vi "Return Stamp.vi"(8 "error in":errorcluster, 10 "Slot Number":i32, 11 "GrabberTool in":refnum<class "GrabberTool Class.lvclass">) -> (0 "error out":errorcluster, 3 "GrabberTool out":refnum<class "GrabberTool Class.lvclass">)   [LabVIEW 2011, in "GrabberTool Class.lvclass"]
uses:
  GrabberTool Class.lvclass
  Config Manager Class/Type Definitions/Named Position.ctl
  Config Manager Class/Type Definitions/Part Type.ctl
  Config Manager Class/Type Definitions/Offset.ctl
  WorkTable Class/WorkTable Class.lvclass
  Vec3d Class/Vec3d Class.lvclass
  Config Manager Class/Config Manager Class.lvclass
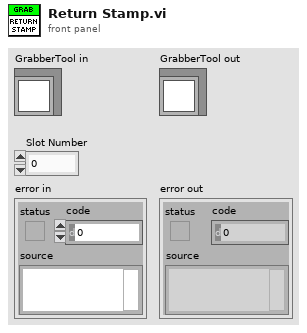
[diagram p1: front panel]
types:
  T1 = typedef "Named Position.ctl" = enum16{"home", "module_chuck_0", "module_chuck_1", "module_chuck_2", "module_chuck_3", "module_chuck_4", "glue_reservoir_chuck", "stamp_tool_chuck", "weight_tool_chuck", "needle_calibration", "tool_rack_pos_0_in", "tool_rack_pos_0_out", "tool_rack_pos_1_in", "tool_rack_pos_1_out", "tool_rack_pos_2_in", "tool_rack_pos_2_out", "front_load_position", "grabber_start_pos", "between_chuck_0_and_1", "between_chuck_2_and_3"}
  T2 = typedef "Part Type.ctl" = enum16{"BBM", "HDI", "BARE HDI", "GLUERESERVOIR", "STAMP_1", "STAMP_2", "STAMP_3", "STAMP_4", "STAMP_5", "WEIGHT_1", "WEIGHT_2", "WEIGHT_3", "WEIGHT_4", "WEIGHT_5", "WEIGHT_6", "WEIGHT_7", "WEIGHT_8", "PICKER_TOOL", "GRABER_TOOL"}
  T3 = typedef "Offset.ctl" = enum16{"needle_offset", "tool_holder_offset"}
  T4 = typedef "Worktable_Stamps.ctl" = cluster{"Stamp Slots":T5[], "Vacuum Channel":i32}
  T5 = typedef "Worktable_Stamp.ctl" = cluster{"Stamp State":enum16{"Empty", "Populated", "Used"}, "Location/Orientation":T6, "Stamp Type":T7}
  T6 = typedef "Position_Orientation.ctl" = cluster{"Center":refnum<class "Vec3d Class.lvclass">, "Orientation":refnum<class "Orient3d Class.lvclass">}
  T7 = typedef "Stamp Type.ctl" = enum16{"Stamp 1", "Stamp 2", "Stamp 3", "Stamp 4", "Stamp 5"}
  T8 = typedef "Gluing Parameters.ctl" = cluster{"Safe Grabber Pickup":dbl, "Safe Grabber Lift":dbl, "Glue Resevoir Wait Time":dbl, "Glue BM Wait Time ":dbl, "Placed Weight X-Move":dbl}
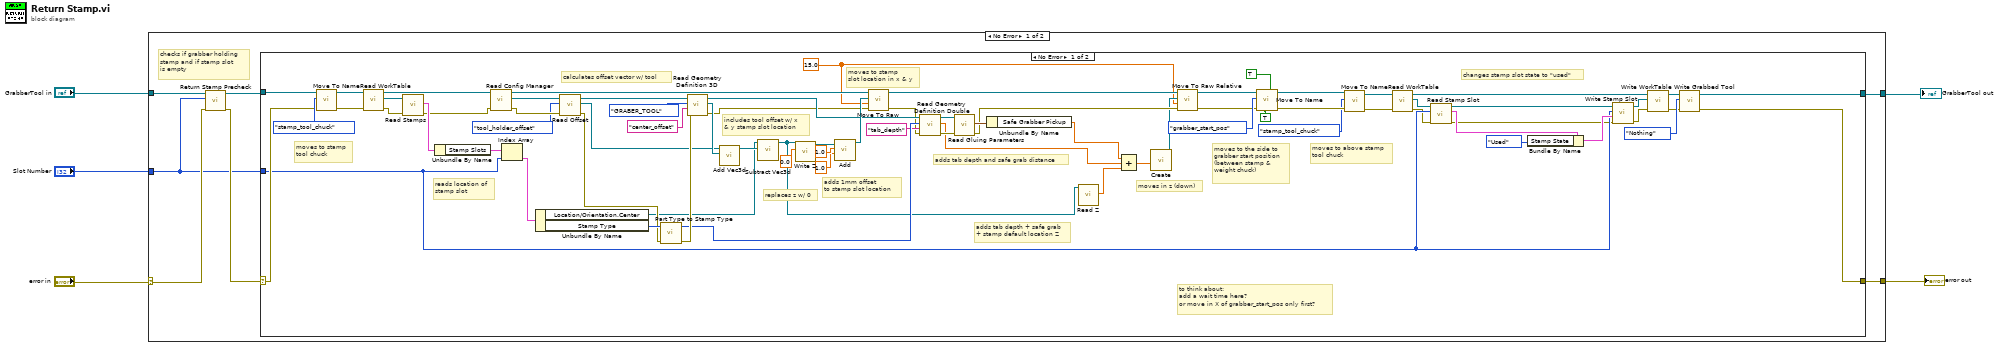
[diagram p0: block diagram]
diagram:
  n1 = case shown="No Error" "error in" {
    selector: "error in" -> [w8 w89]
    tunnel: [w12 w89] -> w5
    tunnel: "GrabberTool in" -> [w10 w90]
    tunnel: "Slot Number" -> [w6 _]
    tunnel: [w11 w90] -> w2
    frame No Error {
      # "checks if grabber holding\nstamp and if stamp slot\nis empty"
      n2 = call "Return Stamp Precheck.vi"("error in (no error)"=w8, "Slot Number"=w6, "GrabberTool Class in"=w10) -> ("error out"=w7:errorcluster, "GrabberTool Class out"=w9:refnum<class "GrabberTool Class.lvclass">)  [unwired: 7 in]
      n3 = case shown="No Error" w7 {
        selector: w7 -> [w83 w88]
        tunnel: [w20 w88] -> w12
        tunnel: w9 -> [w86 w87]
        tunnel: w6 -> [w27 _]
        tunnel: [w21 w87] -> w11
        frame No Error {
          w13 = 15.0 ("Speed")
          # "changes stamp slot state to \"used\""
          # "to think about:\nadd a wait time here?\nor move in X of grabber_start_pos only first?"
          # "moves to above stamp\ntool chuck"
          # "moves to the side to\ngrabber start position\n(between stamp & \nweight chuck)"
          # "moves in z (down)"
          # "adds tab depth + safe grab\n+ stamp default location Z"
          # "adds tab depth and safe grab distance"
          # "moves to stamp\nslot location in x & y"
          # "adds 1mm offset\nto stamp slot location"
          # "includes tool offset w/ x \n& y stamp slot location"
          # "replaces z w/ 0"
          # "calculates offset vector w/ tool"
          # "reads location of\nstamp slot"
          # "moves to stamp\ntool chuck"
          n4 = call-dynamic "Move To Name.vi"("error in"=w83, "Destination"=Named_Position."stamp_tool_chuck", "Gantry in"=w86) -> ("error out"=w82:errorcluster, "Gantry out"=w84:refnum<class "GrabberTool Class.lvclass">)  [unwired: 7 in]
          n5 = call-dynamic "Read WorkTable.vi"("error in"=w82, "Gantry Class in"=w84) -> ("error out"=w80:errorcluster, "WorkTable Class.lvclass"=w81:refnum<class "WorkTable Class.lvclass">, "Gantry Class out"=w76:refnum<class "GrabberTool Class.lvclass">)  [unwired: 7 in]
          n6 = call-dynamic "Read Stamps.vi"("error in (no error)"=w80, "WorkTable Class in"=w81) -> ("error out"=w75:errorcluster, "Stamps"=w79:T4)  [unwired: 7 in, 1 out]
          n7 = Unbundle By Name(w79) -> ("Stamp Slots"=w78:T5[])
          n8 = call-dynamic "Read Config Manager.vi"("error in"=w75, "Gantry in"=w76) -> ("error out"=w73:errorcluster, "Config Manager"=w74:refnum<class "Config Manager Class.lvclass">, "Gantry out"=w62:refnum<class "GrabberTool Class.lvclass">)  [unwired: 7 in]
          n9 = Index Array(array=w78, index=w27) -> (element=w77:T5)
          n10 = Unbundle By Name(w77) -> ("Location/Orientation.Center"=w19:refnum<class "Vec3d Class.lvclass">, "Stamp Type"=w68:T7)
          n11 = call "Read Offset.vi"("error in"=w73, "Offset"=Offset."tool_holder_offset", "Config Manager in"=w74) -> ("error out"=w67:errorcluster, "Vec3d out"=w64:refnum<class "Vec3d Class.lvclass">, "Config Manager out"=w71:refnum<class "Config Manager Class.lvclass">)  [unwired: 6 in]
          n12 = call "Part Type to Stamp Type.vi"("error in"=w67, "Stamp Type"=w68) -> ("error out"=w66:errorcluster, "Part Type"=w56:T2)  [unwired: 8 in]
          n13 = call "Read Geometry Definition 3D.vi"("error in"=w66, "Feature"="center_offset", "Part Type"=Part_Type."GRABER_TOOL", "Config Manager in"=w71) -> ("error out"=w54:errorcluster, "Feature Coordinates"=w65:refnum<class "Vec3d Class.lvclass">, "Config Manager out"=w58:refnum<class "Config Manager Class.lvclass">)  [unwired: 5 in]
          n14 = call-dynamic "Add Vec3d.vi"(10:"Vec3d Class in"=w65, 11:"Vec3d Class in"=w64) -> ("Vec3d Class out"=w40:refnum<class "Vec3d Class.lvclass">)  [unwired: 8 in, 1 out]
          n15 = call "Subtract Vec3d.vi"("Vec3d in 2"=w40, "Vec3d in 1"=w19) -> ("Vec3d Class out"=w18:refnum<class "Vec3d Class.lvclass">)  [unwired: 8 in, 1 out]
          n16 = call-dynamic "Write Z.vi"("Z"=0.0, "Vec3d Class in"=w18) -> ("Vec3d Class out"=w41:refnum<class "Vec3d Class.lvclass">)  [unwired: 8 in, 1 out]
          n17 = call-dynamic "Add.vi"("Y"=1.0, "X"=1.0, "Vec3d in"=w41) -> ("Vec3d out"=w61:refnum<class "Vec3d Class.lvclass">)  [unwired: 6 in, 1 out]
          n18 = call-dynamic "Move To Raw.vi"("error in"=w54, "Speed"=w13, "Destination"=w61, "Gantry in"=w62) -> ("error out"=w53:errorcluster, "Gantry out"=w50:refnum<class "GrabberTool Class.lvclass">)  [unwired: 6 in]
          n19 = call "Read Geometry Definition Double.vi"("error in"=w53, "Feature"="tab_depth", "Part Type"=w56, "Config Manager in"=w58) -> ("error out"=w52:errorcluster, "Geometry Definition"=w38:dbl, "Config Manager out"=w57:refnum<class "Config Manager Class.lvclass">)  [unwired: 5 in]
          n20 = call "Read Gluing Parameters.vi"("error in (no error)"=w52, "Config Manager Class in"=w57) -> ("error out"=w49:errorcluster, "Gluing Parameters"=w51:T8)  [unwired: 7 in, 1 out]
          n21 = Unbundle By Name(w51) -> ("Safe Grabber Pickup"=w39:dbl)
          n22 = call-dynamic "Read Z.vi"("Vec3d Class in"=w18) -> ("Z"=w37:dbl)  [unwired: 8 in, 2 out]
          n23 = Compound Arithmetic op=ADD(w39, w38, w37) -> (w36:dbl)
          n24 = call "Create.vi"("Z"=w36) -> ("Vec3d Class out"=w48:refnum<class "Vec3d Class.lvclass">)  [unwired: 9 in, 1 out]
          n25 = call-dynamic "Move To Raw Relative.vi"("error in"=w49, "Speed(mm/s)"=w13, "Delta"=w48, "Gantry in"=w50) -> ("error out"=w45:errorcluster, "Gantry out"=w47:refnum<class "GrabberTool Class.lvclass">)  [unwired: 6 in]
          n26 = call-dynamic "Move To Name.vi"("Invert"=TRUE, "Direct"=TRUE, "error in"=w45, "Destination"=Named_Position."grabber_start_pos", "Gantry in"=w47) -> ("error out"=w43:errorcluster, "Gantry out"=w44:refnum<class "GrabberTool Class.lvclass">)  [unwired: 5 in]
          n27 = call-dynamic "Move To Name.vi"("error in"=w43, "Destination"=Named_Position."stamp_tool_chuck", "Gantry in"=w44) -> ("error out"=w33:errorcluster, "Gantry out"=w34:refnum<class "GrabberTool Class.lvclass">)  [unwired: 7 in]
          n28 = call-dynamic "Read WorkTable.vi"("error in"=w33, "Gantry Class in"=w34) -> ("error out"=w26:errorcluster, "WorkTable Class.lvclass"=w31:refnum<class "WorkTable Class.lvclass">, "Gantry Class out"=w32:refnum<class "GrabberTool Class.lvclass">)  [unwired: 7 in]
          n29 = call "Read Stamp Slot.vi"("error in (no error)"=w26, "Stamp Slot"=w27, "WorkTable Class in"=w31) -> ("error out"=w25:errorcluster, "Stamp Slot"=w30:T5, "WorkTable Class out"=w29:refnum<class "WorkTable Class.lvclass">)  [unwired: 6 in]
          n30 = Bundle By Name(cluster=w30, "Stamp State"=enum16{"Empty", "Populated", "Used"}."Used") -> (w28:T5)
          n31 = call "Write Stamp Slot.vi"("error in (no error)"=w25, 9:"Stamp Slot"=w28, 10:"Stamp Slot"=w27, "WorkTable Class in"=w29) -> ("error out"=w24:errorcluster, "WorkTable Class out"=w23:refnum<class "WorkTable Class.lvclass">)  [unwired: 6 in]
          n32 = call-dynamic "Write WorkTable.vi"("error in (no error)"=w24, "WorkTable Class.lvclass"=w23, "Gantry Class in"=w32) -> ("error out"=w14:errorcluster, "Gantry Class out"=w15:refnum<class "GrabberTool Class.lvclass">)  [unwired: 7 in]
          n33 = call "Write Grabbed Tool.vi"("error in (no error)"=w14, "Grabbed Tool"=enum16{"Weight Tool", "Stamp Tool", "Nothing"}."Nothing", "GrabberTool Class in"=w15) -> ("error out"=w20:errorcluster, "GrabberTool Class out"=w21:refnum<class "GrabberTool Class.lvclass">)  [unwired: 7 in]
        }
        frame Error {
        }
      }
    }
    frame Error {
    }
  }
  "error out" <- w5
  "GrabberTool out" <- w2
